vi "Xsens Main Process (VISA).vi"(7 "Sys Msg Queue":refnum<queue>, 8 "error in (no error)":errorcluster, 11 "Xsens Enable?":bool) -> (0 "error out":errorcluster)   [LabVIEW 2019]
doc: "This is the RT top level decoder, parser, and data save API for the XSens MTI 710 INS. It contains several subvis that perform the following functions:\n1. Copy measurement data from the VISA serial read message queue\n2. Perform a checksum on the received data\n3. Inspect the data packet, extracting the data types, byte counts, and data payload into an array\n4. Parse the data types and decode the HEX\n5. Save each message to TDMS file(s)\n\n2020 NREL"
uses:
  Globals and Definitions/System Message.ctl
  Globals and Definitions/Serial - Settings.ctl
  <vilib>/Platform/TimedLoop/XDataNode/timing_clust.ctl
  <vilib>/Platform/TimedLoop/XDataNode/nitl_modes.ctl
  <vilib>/Platform/TimedLoop/XDataNode/wakeup.ctl
  Globals and Definitions/Initialization Globals.vi
  Globals and Definitions/RT Globals RD v1.0.vi
  <vilib>/Utility/file.llb/Write Delimited Spreadsheet (string).vi
  <vilib>/Platform/TimedLoop/XDataNode/XDataNode.xnode
  <vilib>/Platform/TimedLoop/XDataNode/XDNodeRunTimeDep.lvlib
panel:
  out "CS Good":bool
  out "All Msg Sizes (Local)":string[](array[string])
  out "Sorted DTs (Local)":string[](array[string])
  # "Please note: This process does not\ncurrently work with XSens data\npackets that are larger than 254\nbytes. \n\nThe MTData2 format uses a single \nbyte to store the message size for \npackets that are 254 bytes or less,\nhowever it uses 2 bytes for larger\npacket sizes. An exception must be\ncreated to handle 2 byte message \nsize cases, since binary parsing \ndepends heavily on counting bytes.\n\n\nMTData2 groups all data by the\nconfigured sample rate and sends \nthose of the same sample rate as \none packet. Message sizes can be \nkept <254 bytes by using multiple \nsample rates."
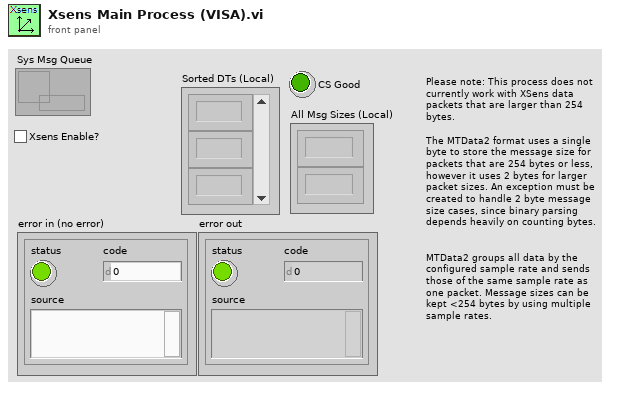
[diagram p1: front panel]
types:
  T1 = typedef "Serial - Settings.ctl" = cluster{"baud rate":u32, "data bits":u16, "parity":enum16{"None", "Odd", "Even", "Mark", "Space"}, "stop bits":u16, "flow control":u16}
  T2 = typedef "XDNodeRunTimeDep.lvlib/timing_clust.ctl" = cluster{"Expected End [f-1]":u64, "Actual End [f-1]":u64, "Finished Late? [f-1]":bool, "Expected End [i-1]":u64, "Actual End [i-1]":u64, "Finished Late? [i-1]":bool, "Expected Start [i]":u64, "Actual Start [i]":u64, "Expected Start [f]":u64, "Actual Start [f]":u64, "Source Name":string, "Structure Name":string, "Period":i64, "Deadline":i64, "Offset":i64, "Start":i64, "Priority":i32, "Timeout":i32, "Mode":T3, "Wakeup Reason":T4, "Error":errorcluster, "Source Type":string, "Secondary Source Type":string, "Global End Time":u64, "Global Start Time":u64, "Frame Duration":u64, "Iteration Duration":u64, "Assigned CPU":i32, "I/O Scan Engine Mode":u32}
  T3 = typedef "XDNodeRunTimeDep.lvlib/nitl_modes.ctl" = enum32{"No Change", "Process missed periods, maintain original phase", "Discard missed periods, maintain original phase", "Process missed periods, ignore original phase", "Discard missed periods, ignore original phase"}
  T4 = typedef "XDNodeRunTimeDep.lvlib/wakeup.ctl" = enum32{"Normal", "Aborted", "Asynchronous wakeup", "Timing source error", "Timed loop error", "Timeout"}
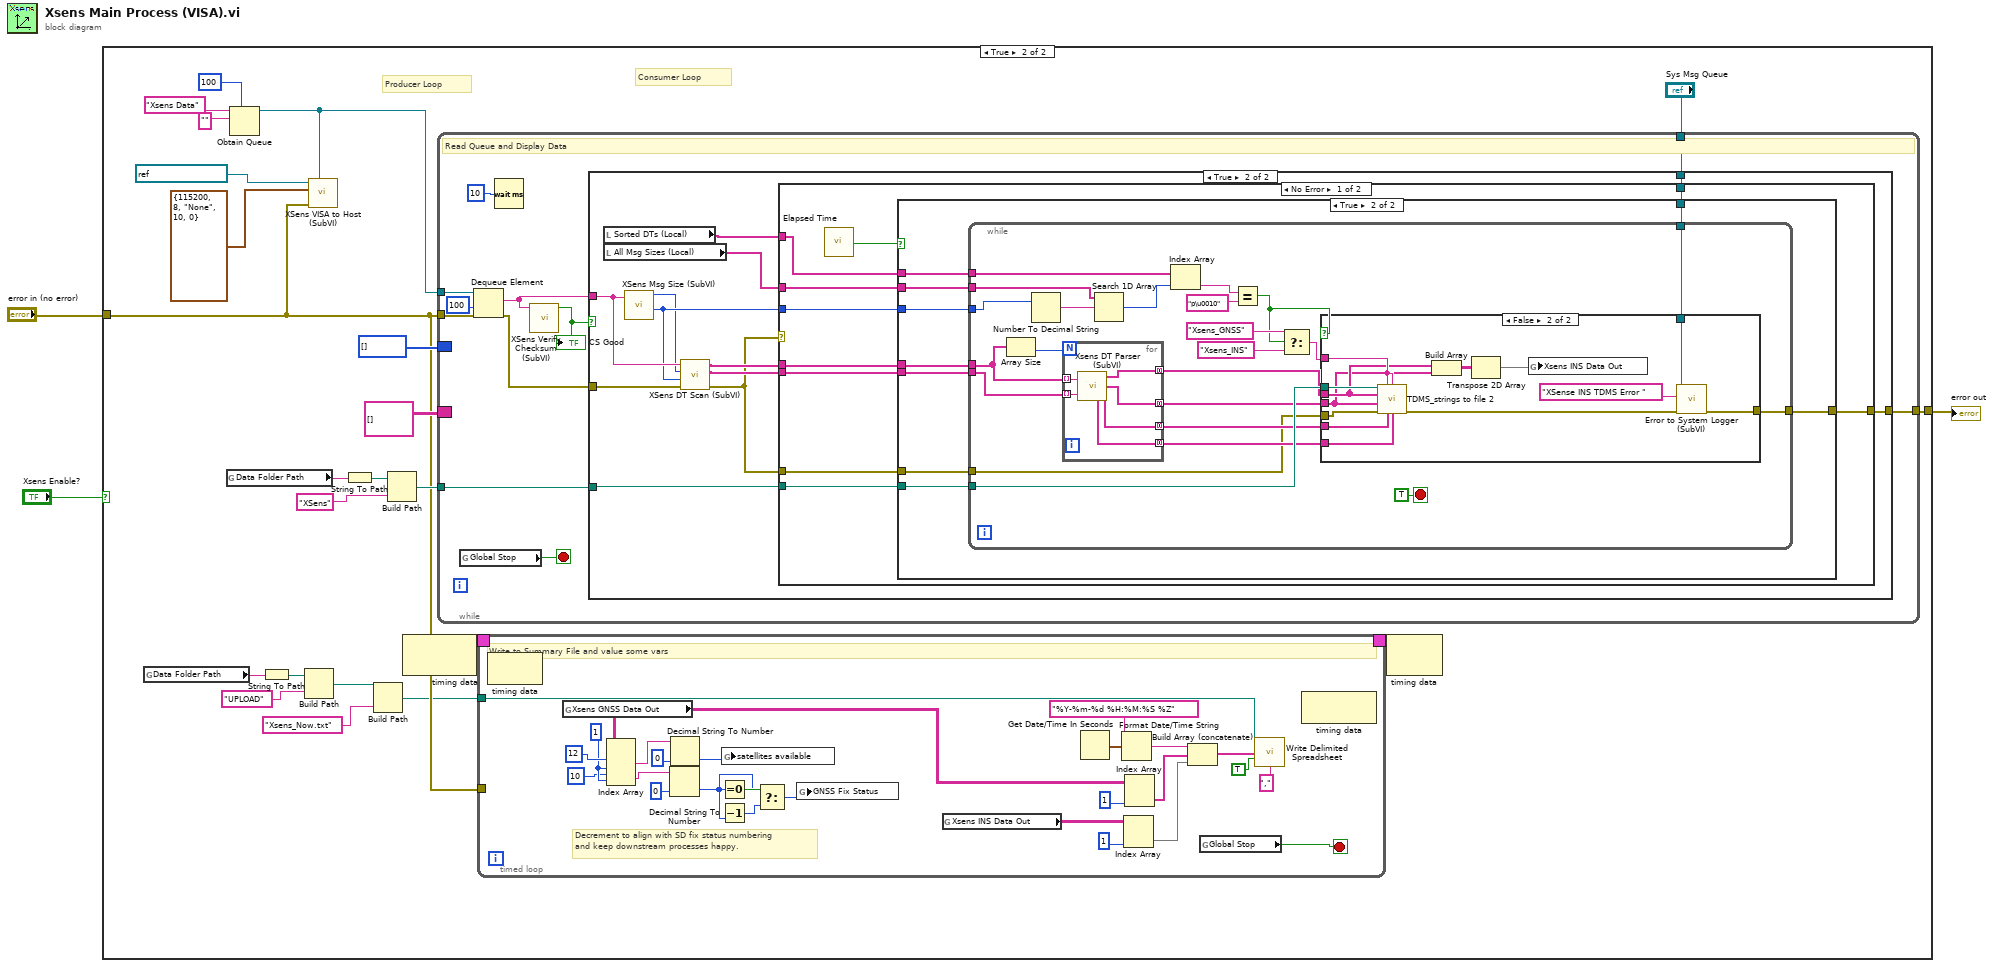
[diagram p0: block diagram]
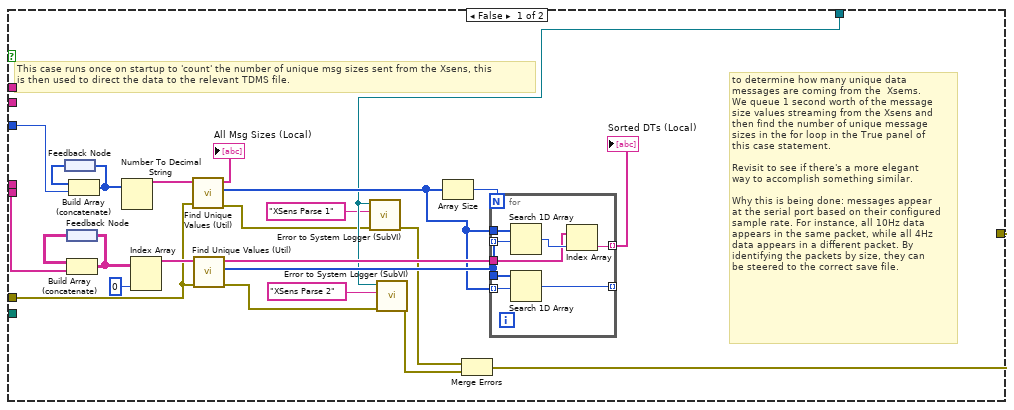
[diagram p4: hidden frame]
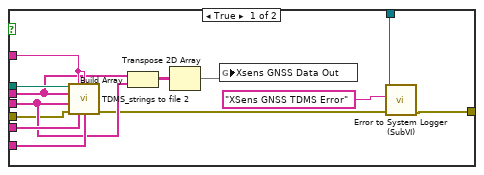
[diagram p5: hidden frame]
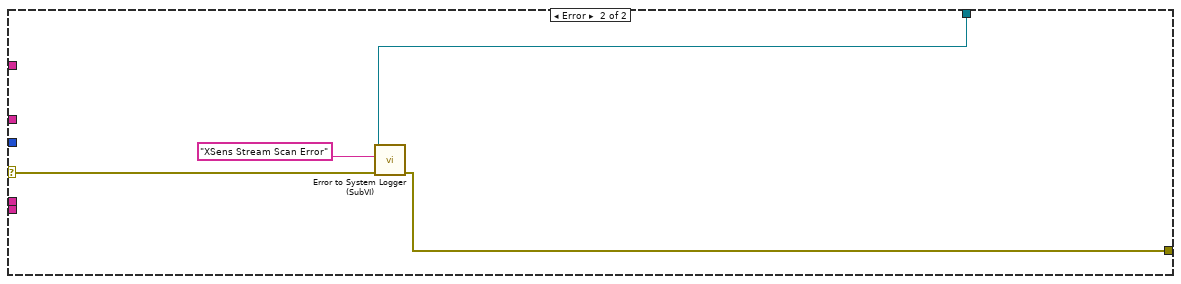
[diagram p6: hidden frame]
diagram:
  n1 = case shown="True" "Xsens Enable?" {
    tunnel: [w4 w16] -> w3
    tunnel: "error in (no error)" -> [w4 w6]
    frame False {
    }
    frame True {
      # "Consumer Loop"
      # "Producer Loop"
      n2 = global read "Initialization Globals.vi" "Data Folder Path"() -> (w9:string)
      n3 = global read "Initialization Globals.vi" "Data Folder Path"() -> (w21:string)
      n4 = Obtain Queue(max queue size (-1, unlimited)=100, name (unnamed)="Xsens Data", element data type="") -> (queue out=w14:refnum<queue>)  [unwired: 2 in, 2 out]
      n5 = String To Path(string=w9) -> (path=w10:path)
      n6 = Build Path(base path=w10, name or relative path="UPLOAD") -> (appended path=w7:path)
      n7 = call "XSens VISA to Host (SubVI).vi"("XSense Queue In"=w14, "error in (no error)"=w6, "Serial Settings"=T1 {"baud rate"=115200, "data bits"=8, "parity"=enum."None", "stop bits"=10, "flow control"=0}, "VISA resource name"=refnum<visa-resource-name> "ASRL3::INSTR") -> ()  [unwired: 7 in, 1 out]
      n8 = String To Path(string=w21) -> (path=w22:path)
      n9 = Build Path(base path=w7, name or relative path="Xsens_Now.txt") -> (appended path=w5:path)
      n10 = Build Path(base path=w22, name or relative path="XSens") -> (appended path=w20:path)
      n11 = node-c288() -> (w27:T2)  [unwired: 1 in]
      n12 = while {
        tunnel: w20 -> [w66]
        border: string[][] [] -> [_]
        border: u16[] [] -> [_]
        tunnel: w14 -> [w65]
        tunnel: w6 -> [w62]
        tunnel: "Sys Msg Queue" -> [w60]
        tunnel: [w59] -> w16
        stop <- w58 stop-if-true
        # "Read Queue and Display Data"
        n13 = global read "RT Globals RD v1.0.vi" "Global Stop"() -> (w58:bool)
        n14 = Dequeue Element(queue=w65, timeout in ms (-1)=100, error in (no error)=w62) -> (element=w64:string, error out=w61:errorcluster)  [unwired: 2 out]
        n15 = Wait (ms)(milliseconds to wait=u32 10) -> ()  [unwired: 1 out]
        n16 = call "XSens Verify Checksum (SubVI).vi"("MTData2 Msg"=w64) -> ("CS Good?"=w67:bool)  [unwired: 10 in]
        "CS Good" <- w67
        n17 = case shown="True" w67 {
          tunnel: w64 -> [_ w78]
          tunnel: w66 -> [_ w81]
          tunnel: w61 -> [w69 w75]
          tunnel: w60 -> [_ w80]
          tunnel: [w69 w79] -> w59
          frame False {
          }
          frame True {
            n18 = local read "Sorted DTs (Local)"() -> (w71:string[])
            n19 = local read "All Msg Sizes (Local)"() -> (w70:string[])
            n20 = call "XSens Msg Size (SubVI).vi"("From Q"=w78) -> ("Data Size"=w73:u16, "Index"=w72:i16)  [unwired: 9 in]
            n21 = call "XSens DT Scan (SubVI).vi"("string in"=w78, "Index"=w72, "Payload Size"=w73, "Error In"=w75) -> ("DT Out"=w77:string[], "DT String"=w76:string[], "Error Out"=w74:errorcluster)  [unwired: 2 in]
            n22 = case shown="No Error" w74 {
              selector: w74 -> [_ w191]
              tunnel: w81 -> [w90 _]
              tunnel: w74 -> [w89 _]
              tunnel: w80 -> [w88 w188]
              tunnel: [w87 w190] -> w79
              tunnel: w77 -> [w86 _]
              tunnel: w76 -> [w85 _]
              tunnel: w73 -> [w84 _]
              tunnel: w71 -> [w83 _]
              tunnel: w70 -> [w82 _]
              frame No Error {
                n23 = call "Elapsed Time"() -> ("Time has Elapsed"=w91:bool)  [unwired: 12 in, 7 out]
                n24 = case shown="True" w91 {
                  tunnel: w86 -> [w105 w132]
                  tunnel: w85 -> [_ w131]
                  tunnel: w84 -> [w113 w130]
                  tunnel: w90 -> [_ w129]
                  tunnel: w89 -> [w94 w128]
                  tunnel: w88 -> [w96 w127]
                  tunnel: [w98 w126] -> w87
                  tunnel: w83 -> [_ w125]
                  tunnel: w82 -> [_ w124]
                  frame False {
                    # "This case runs once on startup to 'count' the number of unique msg sizes sent from the Xsens, this\nis then used to direct the data to the relevant TDMS file."
                    # "to determine how many unique data\nmessages are coming from the  Xsems.\nWe queue 1 second worth of the message\nsize values streaming from the Xsens and\nthen find the number of unique message\nsizes in the for loop in the True panel of \nthis case statement. \n\nRevisit to see if there's a more elegant \nway to accomplish something similar.\n\nWhy this is being done: messages appear\nat the serial port based on their configured\nsample rate. For instance, all 10Hz data\nappears in the same packet, while all 4Hz\ndata appears in a different packet. By \nidentifying the packets by size, they can \nbe steered to the correct save file."
                    n25 = feedback #1() -> (w112:u16[])
                    n26 = feedback #2() -> (w115:string[][])
                    n27 = Build Array (concatenate)(w115, w105) -> (w104:string[][])
                    n28 = feedback-in #2(w104) -> ()
                    n29 = Build Array (concatenate)(w112, w113) -> (w111:u16[])
                    n30 = feedback-in #1(w111) -> ()
                    n31 = Number To Decimal String(number=w111) -> (decimal integer string=w103:string[])  [unwired: 1 in]
                    n32 = Index Array(array=w104, index (col)=0 ("disabled index (col)")) -> (element=w106:string[])  [unwired: 1 in]
                    n33 = call "Find Unique Values (Util).vi"("error in (no error)"=w94, "Array in"=w103) -> ("error out"=w93:errorcluster, "Number repeats for each"=w101:i32[], "Unique Values"=→"All Msg Sizes (Local)":string[])  [unwired: 7 in]
                    n34 = call "Find Unique Values (Util).vi"("error in (no error)"=w94, "Array in"=w106) -> ("error out"=w92:errorcluster, "Number repeats for each"=w109:i32[], "Unique Values"=w108:string[])  [unwired: 7 in]
                    n35 = call "Error to System Logger (SubVI).vi"("error in (no error)"=w93, "Message Tag"="XSens Parse 1", "Sys Msg Queue"=w96) -> ("error out"=w100:errorcluster)  [unwired: 8 in]
                    n36 = call "Error to System Logger (SubVI).vi"("error in (no error)"=w92, "Message Tag"="XSens Parse 2", "Sys Msg Queue"=w96) -> ("error out"=w99:errorcluster)  [unwired: 8 in]
                    n37 = Array Size(array=w101) -> (size(s)=w110:i32)
                    n38 = Merge Errors(w100, w99) -> (w98:errorcluster)
                    n39 = for {
                      N: w110 -> [_]
                      tunnel: w101 -> [w123]
                      tunnel: w109 -> [w122]
                      tunnel: w101 -> [w121] mode=indexing
                      tunnel: w109 -> [w120] mode=indexing
                      tunnel: [w119] -> _ mode=indexing
                      tunnel: w108 -> [w117]
                      tunnel: [w116] -> w107 mode=indexing
                      n40 = Search 1D Array(1D array=w123, element=w120) -> (index of element=w118:i32)  [unwired: 1 in]
                      n41 = Search 1D Array(1D array=w122, element=w121) -> (index of element=w119:i32)  [unwired: 1 in]
                      n42 = Index Array(array=w117, index=w118) -> (element=w116:string)
                    }
                    "Sorted DTs (Local)" <- w107
                  }
                  frame True {
                    n43 = while {
                      tunnel: w132 -> [w155]
                      tunnel: w131 -> [w154]
                      tunnel: w130 -> [w146]
                      tunnel: w129 -> [w151]
                      tunnel: w128 -> [w137]
                      tunnel: [w136] -> w126
                      tunnel: w127 -> [w135]
                      tunnel: w125 -> [w134]
                      tunnel: w124 -> [w133]
                      stop <- TRUE stop-if-true
                      n44 = Array Size(array=w155) -> (size(s)=w152:i32)
                      n45 = Number To Decimal String(number=w146) -> (decimal integer string=w145:string)  [unwired: 1 in]
                      n46 = for {
                        N: w152 -> [_]
                        tunnel: w155 -> [w187] mode=indexing
                        tunnel: w154 -> [w186] mode=indexing
                        tunnel: [w184] -> w149 mode=concatenating
                        tunnel: [w185] -> w150 mode=concatenating
                        tunnel: [w183] -> w148 mode=concatenating
                        tunnel: [w182] -> w147 mode=concatenating
                        n47 = call "Xsens DT Parser (SubVI).vi"("DT String In"=w186, "DataType In"=w187) -> ("Channel Units"=w183:string[], "Channel DataTypes"=w182:string[], "Decoded Data Out"=w184:string[], "Channel Names"=w185:string[])  [unwired: 1 in]
                      }
                      n48 = Search 1D Array(1D array=w133, element=w145) -> (index of element=w144:i32)  [unwired: 1 in]
                      n49 = Index Array(array=w134, index=w144) -> (element=w142:string)
                      n50 = Equal?(x=w142, y="p\u0010") -> (x = y?=w138:bool)
                      n51 = Select(t="Xsens_GNSS" ("group name"), s=w138, f="Xsens_INS" ("group name")) -> (s? t:f=w139:string)
                      n52 = case shown="False" w138 {
                        tunnel: w151 -> [w168 w181]
                        tunnel: w150 -> [w163 w177]
                        tunnel: w149 -> [w162 w176]
                        tunnel: w148 -> [w167 w180]
                        tunnel: w147 -> [w166 w179]
                        tunnel: w139 -> [w165 w178]
                        tunnel: w137 -> [w161 w174]
                        tunnel: [w159 w172] -> w136
                        tunnel: w135 -> [w160 w170]
                        frame True {
                          n53 = call "TDMS_strings to file 2.vi"("Base path"=w168, "Group Name"=w165, "FileName"=w165, "Channel Names"=w163, "Data"=w162, "error in (no error)"=w161, "Channel Units"=w167, "property Metadata"=w166) -> ("error out"=w158:errorcluster)  [unwired: 6 in, 1 out]
                          n54 = Build Array(w163, w162) -> (w164:string[][])
                          n55 = Transpose 2D Array(2D array=w164) -> (transposed array=w156:string[][])
                          n56 = global write "RT Globals RD v1.0.vi" "Xsens GNSS Data Out"(w156) -> ()
                          n57 = call "Error to System Logger (SubVI).vi"("error in (no error)"=w158, "Message Tag"="XSens GNSS TDMS Error", "Sys Msg Queue"=w160) -> ("error out"=w159:errorcluster)  [unwired: 8 in]
                        }
                        frame False {
                          n58 = call "TDMS_strings to file 2.vi"("Base path"=w181, "Group Name"=w178, "FileName"=w178, "Channel Names"=w177, "Data"=w176, "error in (no error)"=w174, "Channel Units"=w180, "property Metadata"=w179) -> ("error out"=w173:errorcluster)  [unwired: 6 in, 1 out]
                          n59 = Build Array(w177, w176) -> (w175:string[][])
                          n60 = Transpose 2D Array(2D array=w175) -> (transposed array=w169:string[][])
                          n61 = global write "RT Globals RD v1.0.vi" "Xsens INS Data Out"(w169) -> ()
                          n62 = call "Error to System Logger (SubVI).vi"("error in (no error)"=w173, "Message Tag"="XSense INS TDMS Error ", "Sys Msg Queue"=w170) -> ("error out"=w172:errorcluster)  [unwired: 8 in]
                        }
                      }
                    }
                  }
                }
              }
              frame Error {
                n63 = call "Error to System Logger (SubVI).vi"("error in (no error)"=w191, "Message Tag"="XSens Stream Scan Error", "Sys Msg Queue"=w188) -> ("error out"=w190:errorcluster)  [unwired: 8 in]
              }
            }
          }
        }
      }
      n64 = timed-loop {
        timing: w27 -> [_]
        timing-out: [_] -> w26
        tunnel: w6 -> [_]
        tunnel: w5 -> [w34]
        stop <- w51 stop-if-true
        w50 = 1 ("disabled index (col)")
        # "Decrement to align with SD fix status numbering\nand keep downstream processes happy."
        # "Write to Summary File and value some vars"
        n65 = node-c288() -> ()  [unwired: 1 in, 1 out]
        n66 = global read "RT Globals RD v1.0.vi" "Xsens GNSS Data Out"() -> (w33:string[][])
        n67 = Index Array(array=w33, index (row) #1=12 ("index (row)"), index (col) #1=w50, index (row) #2=10 ("disabled index (row)"), index (col) #2=w50) -> (element #1=w52:string, element #2=w45:string)
        n68 = Decimal String To Number(string=w45, default (0L)=u32 0 ("default (0 I32)")) -> (number=w44:u32)  [unwired: 1 in, 1 out]
        n69 = Decimal String To Number(string=w52, default (0L)=u8 0 ("default (0 I32)")) -> (number=w46:u8)  [unwired: 1 in, 1 out]
        n70 = Equal To 0?(x=w44) -> (x = 0?=w48:bool)
        n71 = Decrement(x=w44) -> (x-1=w47:u32)
        n72 = global write "RT Globals RD v1.0.vi" "satellites available"(w46) -> ()
        n73 = Select(t=w44, s=w48, f=w47) -> (s? t:f=w43:u32)
        n74 = global write "RT Globals RD v1.0.vi" "GNSS Fix Status"(w43) -> ()
        n75 = global read "RT Globals RD v1.0.vi" "Xsens INS Data Out"() -> (w30:string[][])
        n76 = Get Date/Time In Seconds() -> (seconds since 1Jan1904=w39:timestamp)
        n77 = Format Date/Time String(time format string (%c)="%Y-%m-%d %H:%M:%S %Z", seconds (now)=w39) -> (date/time string=w38:string)  [unwired: 1 in]
        n78 = Index Array(array=w30, index (col)=1 ("index")) -> (element=w29:string[])  [unwired: 1 in]
        n79 = Index Array(array=w33, index (col)=1 ("index")) -> (element=w31:string[])  [unwired: 1 in]
        n80 = Build Array (concatenate)(w38, w31, w29) -> (w35:string[])
        n81 = global read "RT Globals RD v1.0.vi" "Global Stop"() -> (w51:bool)
        n82 = call-poly <vilib>:"Write Delimited Spreadsheet.vi"("file path (dialog if empty)"=w34, "1D data"=w35, "append to file? (new file:F)"=TRUE, "delimiter (\\t)"="," ("delimiter (\\t)")) -> ()  [unwired: 10 in, 2 out]
        n83 = node-c288() -> ()  [unwired: 1 in, 1 out]
      }
      n84 = node-c288(w26) -> ()  [unwired: 1 out]
    }
  }
  "error out" <- w3
